vi "Insert Wrap.vi"(10 "Msg":refnum<class "Msg.lvclass">, 11 "TEMPLATE Actor in":refnum<class "TEMPLATE Actor.lvclass">) -> (3 "TEMPLATE Actor out":refnum<class "TEMPLATE Actor.lvclass">)   [LabVIEW 2020, in "_Template.lvlib" / "Templates.lvlib" / "TEMPLATE Actor.lvlib" / "TEMPLATE Actor.lvclass"]
uses:
  TEMPLATE Actor.lvclass
  C:/git/jettl/src/jettl/jettl/Actor/Actor/Actor.lvclass
  jettl/jettl/Msg/Msg.lvclass
  TEMPLATE Actor.lvclass/TEMPLATE Actor.ctl
  jettl/jettl/Attributes/Attributes/Attributes.lvclass
  jettl/jettl/Actor/Actor/Actor.lvclass
  jettl/jettl/Actor/Actor.lvlib
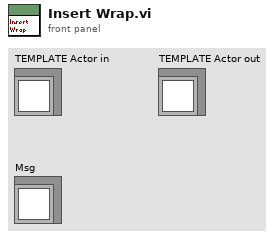
[diagram p1: front panel]
types:
  T1 = typedef "jettl.lvlib/Actor.lvlib/Msgs.ctl" = set{refnum<class "Msg.lvclass">}
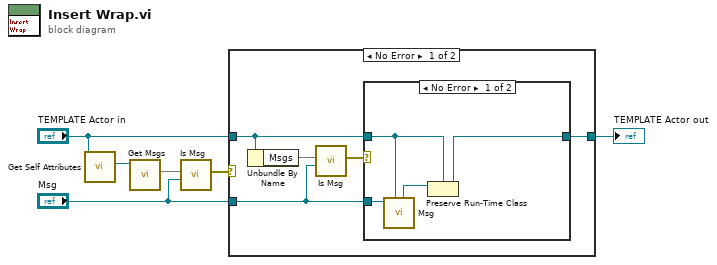
[diagram p0: block diagram]
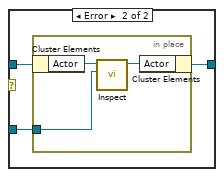
[diagram p2: hidden frame]
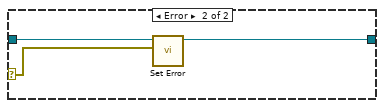
[diagram p3: hidden frame]
diagram:
  n1 = call-dynamic "Get Self Attributes.vi"("TEMPLATE Actor in"="TEMPLATE Actor in") -> ("Self Attributes"=w6:refnum<class "Attributes.lvclass">)  [unwired: 10 in]
  n2 = call-dynamic "Get Msgs.vi"("Attributes in"=w6) -> ("Msgs"=w5:T1)  [unwired: 10 in]
  n3 = call "Is Msg.vi"("Msg"="Msg", "Msgs"=w5) -> ("Error"=w4:errorcluster)  [unwired: 9 in]
  n4 = case shown="No Error" w4 {
    selector: w4 -> [_ w22]
    tunnel: [w9 w23] -> w2
    tunnel: "TEMPLATE Actor in" -> [w8 w24]
    tunnel: "Msg" -> [w7 _]
    frame No Error {
      n5 = Unbundle By Name(w8) -> ("Msgs"=w11:T1)
      n6 = call "Is Msg.vi"("Msg"=w7, "Msgs"=w11) -> ("Error"=w10:errorcluster)  [unwired: 9 in]
      n7 = case shown="No Error" w10 {
        tunnel: w8 -> [w13 w18]
        tunnel: [w12 w17] -> w9
        tunnel: w7 -> [w15 w16]
        frame No Error {
          n8 = call-dynamic "Msg.vi"("Actor in"=w13, "Msg in"=w15) -> ("Actor out"=w14:refnum<class "Actor.lvclass">)  [unwired: 9 in]
          n9 = Preserve Run-Time Class(object in=w14, 2:w13) -> (object out=w12:refnum<class "TEMPLATE Actor.lvclass">)  [unwired: 1 in, 1 out]
        }
        frame Error {
          n10 = in-place {
            in-place-border: w16 -> [w19]
            n11 = in-place-cluster #1(w18) -> ("Actor"=w21:refnum<class "Actor.lvclass">)
            n12 = call-dynamic "Inspect.vi"("Msg"=w19, "Actor in"=w21) -> ("Actor out"=w20:refnum<class "Actor.lvclass">)  [unwired: 9 in]
            n13 = in-place-cluster #1("Actor"=w20) -> (w17:refnum<class "TEMPLATE Actor.lvclass">)
          }
        }
      }
    }
    frame Error {
      n14 = call-dynamic "Set Error.vi"("Error"=w22, "TEMPLATE Actor in"=w24) -> ("TEMPLATE Actor out"=w23:refnum<class "TEMPLATE Actor.lvclass">)  [unwired: 9 in]
    }
  }
  "TEMPLATE Actor out" <- w2
